vi "my UDP Sender.vi"() -> ()   [LabVIEW 2014]
panel:
  out "数组 4":dbl[][](array[numeric])
  out "波形图":dbl[][](graph)
  out "error out":errorcluster caption="错误输出"
  in  "stop (F)":bool caption="停止(F)"
  in  "采样率":i32[](array[numeric])
  in  "timeout (s)":dbl=10.0 caption="超时(s)" format="%0.2f"
  in  "设备名":tag="PXI1Slot2"
  in  "停止":bool
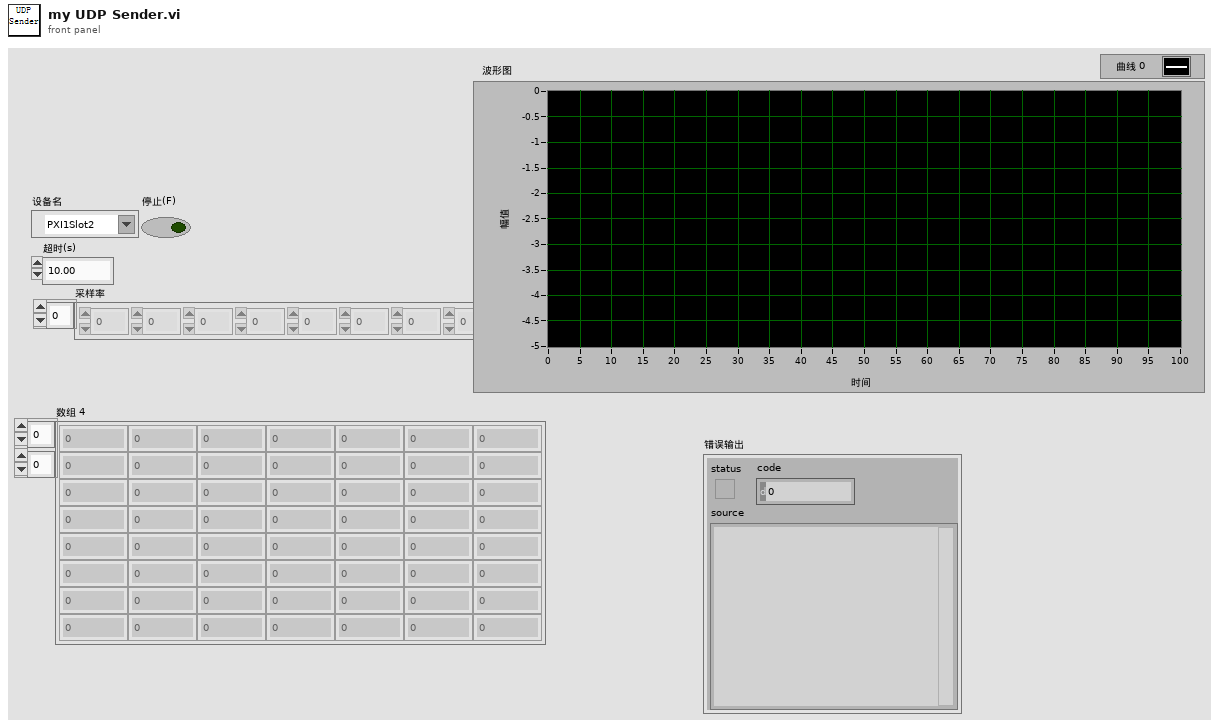
[diagram p1: front panel]
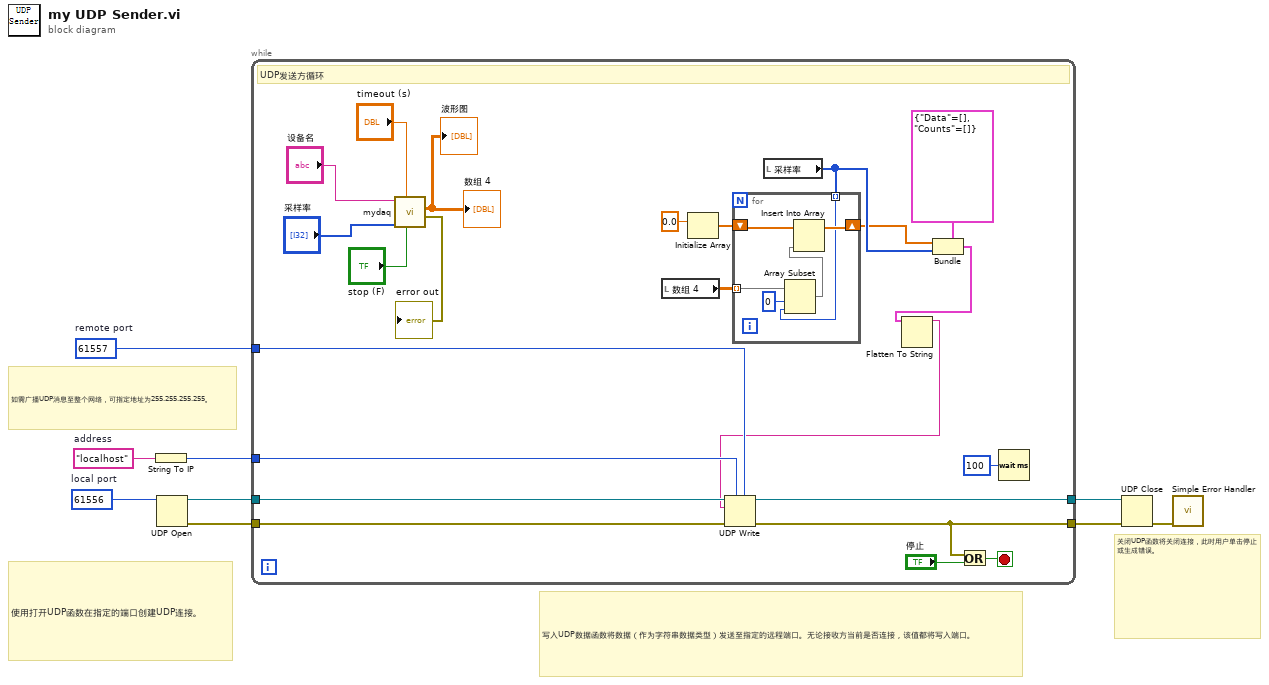
[diagram p0: block diagram]
diagram:
  w1 = u16 61557  # remote port
  w2 = u16 61556  # local port
  w7 = "localhost"  # address
  # "如需广播UDP消息至整个网络，可指定地址为255.255.255.255。"
  # "关闭UDP函数将关闭连接，此时用户单击停止或生成错误。"
  # "写入UDP数据函数将数据（作为字符串数据类型）发送至指定的远程端口。无论接收方当前是否连接，该值都将写入端口。"
  # "使用打开UDP函数在指定的端口创建UDP连接。"
  n1 = String To IP(1:w7) -> (0:w5:u32)
  n2 = UDP Open(11:w2) -> (port=w4:refnum<k16>, 0:w3:errorcluster)  [unwired: 4 in, 1 out]
  n3 = while {
    tunnel: [w27] -> w8
    tunnel: w4 -> [w32]
    tunnel: w3 -> [w31]
    tunnel: [w28] -> w9
    tunnel: w5 -> [w26]
    tunnel: w1 -> [w24]
    stop <- w30 stop-if-true
    # "UDP发送方循环"
    n4 = call "mydaq.vi"("stop (F)"="stop (F)", "timeout (s)"="timeout (s)", "采样率"="采样率", "设备名"="设备名") -> ("error out"=→"error out":errorcluster, "数组 4"=→"波形图" →"数组 4":dbl[][])  [unwired: 6 in]
    n5 = local read "数组 4"() -> (w23:dbl[][])
    n6 = Initialize Array(0.0 ("元素")) -> (w22:dbl[])  [unwired: 1 in]
    n7 = local read "采样率"() -> (w19:i32[])
    n8 = for {
      tunnel: w23 -> [w36] mode=indexing
      shift-right: [w37] -> w10
      shift-left: w22 -> [w38]
      tunnel: w19 -> [w33] mode=indexing
      n9 = Array Subset(array=w36, index=0 ("索引"), length=w33) -> (w35:dbl[])
      n10 = Insert Into Array(array=w38, new element=w35) -> (w37:dbl[])  [unwired: 1 in]
    }
    n11 = Bundle(cluster=cluster{"Data":dbl[], "Counts":i32[]} {"Data"=[], "Counts"=[]}, "Data"=w10, "Counts"=w19) -> (w18:cluster{"Data":dbl[], "Counts":i32[]})
    n12 = Flatten To String(anything=w18) -> (data string=w17:string)  [unwired: 3 in, 2 out]
    n13 = UDP Write(address=w26, port or service name=w24, connection ID=w32, data in=w17, 8:w31) -> (error out=w27:errorcluster, 3:w28:refnum<k16>)  [unwired: 1 in]
    n14 = Or(x=w27, y="停止") -> (x .or. y?=w30:bool)
    n15 = Wait (ms)(milliseconds to wait=u32 100) -> ()  [unwired: 1 out]
  }
  n16 = UDP Close(connection ID=w9, 8:w8) -> (error out=w6:errorcluster)  [unwired: 1 out]
  n17 = call <vilib>:"Simple Error Handler.vi"("error in (no error)"=w6) -> ()  [unwired: 4 in, 5 out]
